vi "To String Array.vi"(8 "error in (no error)":errorcluster, 11 "Conditional Jump Step Config in":refnum<class "Conditional Jump Step Config.lvclass">) -> (0 "error out":errorcluster, 1 "Step String Array":string[](array[string]), 3 "Conditional Jump Step Config out":refnum<class "Conditional Jump Step Config.lvclass">)   [LabVIEW 2015, in "Conditional Jump Step Config.lvclass"]
uses:
  Conditional Jump Step Config.lvclass
  <vilib>/NI/Tag Bus/tag/tag descriptor.lvclass/tag descriptor.ctl
  <vilib>/NI/Tag Bus Module Framework/channel/TBM channel.lvclass
  classes/Step/Config/Step Config.lvclass
  <vilib>/NI/Tag Bus/tag/tag descriptor.lvclass
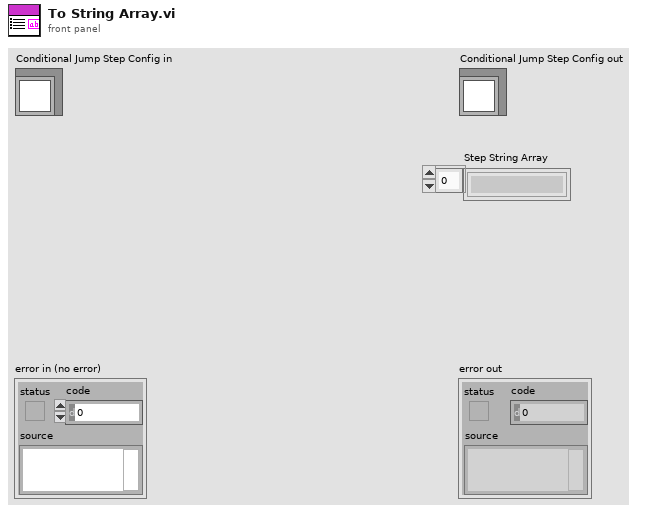
[diagram p1: front panel]
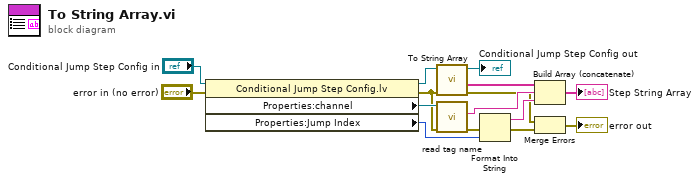
[diagram p0: block diagram]
diagram:
  n1 = property class="Conditional Jump Step Config.lv"(reference="Conditional Jump Step Config in", error in="error in (no error)") -> (reference out=w5:refnum<class "Conditional Jump Step Config.lvclass">, error out=w2:errorcluster, "Properties:channel"=w10:refnum<class "TBM channel.lvclass">, "Properties:Jump Index"=w9:i32)
  n2 = call-parent "To String Array.vi"("error in (no error)"=w2, "Step Config in"=w5) -> ("error out"=w1:errorcluster, "Step String Array"=w3:string[], "Step Config out"=→"Conditional Jump Step Config out":refnum<class "Conditional Jump Step Config.lvclass">)  [unwired: 7 in]
  n3 = call <vilib>:"read tag name.vi"("error in"=w2, "system tag in"=w10) -> ("error out"=w7:errorcluster, "name"=w13:string)  [unwired: 7 in, 1 out]
  n4 = Format Into String(error in=w7, w9) -> (resulting string=w12:string, error out=w8:errorcluster)  [unwired: 2 in]
  n5 = Build Array (concatenate)(w3, w13, w12) -> (→"Step String Array":string[])
  n6 = Merge Errors(w1, w8) -> (→"error out":errorcluster)
